vi "apply modification.vi"(10 "vis":refnum<vi>[](array[refnum]), 11 "reset to origin in":refnum<class "reset to origin.lvclass">) -> (0 "error report":errorcluster[](array[cluster]), 3 "reset to origin out":refnum<class "reset to origin.lvclass">)   [LabVIEW 2013, in "reset to origin.lvclass"]
uses:
  reset to origin.lvclass
  <vilib>/Utility/miscctls.llb/LVPointTypeDef.ctl
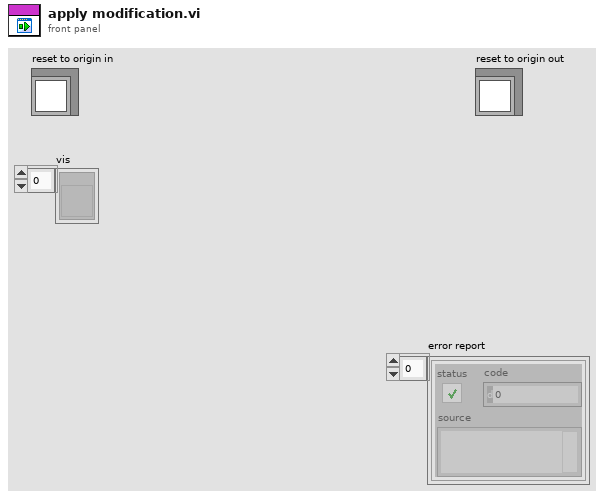
[diagram p1: front panel]
types:
  T1 = typedef "LVPointTypeDef.ctl" = cluster{"Horizontal":i16, "Vertical":i16}
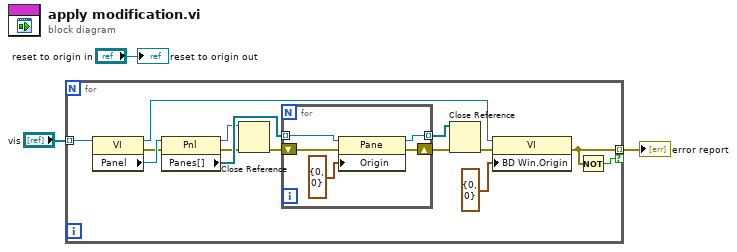
[diagram p0: block diagram]
diagram:
  n1 = for {
    tunnel: "vis" -> [w17] mode=indexing
    tunnel: [w5] -> w1 mode=indexing if=w4
    n2 = property class="VI"(reference=w17) -> (reference out=w6:refnum<vi>, error out=w14:errorcluster, "Panel"=w15:refnum<vi>)  [unwired: 1 in]
    n3 = property class="Pnl"(reference=w15, error in=w14) -> (reference out=w10:refnum<vi>, error out=w11:errorcluster, "Panes[]"=w16:refnum<vi>[])
    n4 = Close Reference(reference=w10, error in (no error)=w11) -> (error out=w9:errorcluster)
    n5 = for {
      tunnel: w16 -> [w22] mode=indexing
      shift-right: [w19] -> w13
      shift-left: w9 -> [w20]
      tunnel: [w18] -> w12 mode=indexing
      n6 = property class="Pane"(reference=w22, error in=w20, "Origin"=T1 {"Horizontal"=0, "Vertical"=0}) -> (reference out=w18:refnum<vi>, error out=w19:errorcluster)
    }
    n7 = Close Reference(reference=w12, error in (no error)=w13) -> (error out=w7:errorcluster)
    n8 = property class="VI"(reference=w6, error in=w7, "BD Win.Origin"=T1 {"Horizontal"=0, "Vertical"=0} ("Origin")) -> (error out=w5:errorcluster)  [unwired: 1 out]
    n9 = Not(x=w5) -> (.not. x?=w4:bool)
  }
  "error report" <- w1
  "reset to origin out" <- "reset to origin in"
